vi "动态调用（非模式对话框）串口基本配置对话框.vi"() -> ()   [LabVIEW 2013]
uses:
  <vilib>/Platform/TimedLoop/XDataNode/timing_clust.ctl
  <vilib>/Platform/TimedLoop/XDataNode/nitl_modes.ctl
  <vilib>/Platform/TimedLoop/XDataNode/wakeup.ctl
  <vilib>/Platform/TimedLoop/XDataNode/XDataNode.xnode
  <vilib>/Platform/TimedLoop/XDataNode/XDNodeRunTimeDep.lvlib
panel:
  out "错误输出":errorcluster
  out "应用程序:所有内存中的VI":string[](array[string])
  in  "串口基本配置对话框":bool
  in  "停止":bool
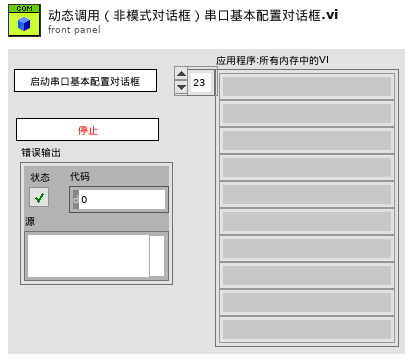
[diagram p1: front panel]
types:
  T1 = typedef "XDNodeRunTimeDep.lvlib/timing_clust.ctl" = cluster{"Expected End [f-1]":u64, "Actual End [f-1]":u64, "Finished Late? [f-1]":bool, "Expected End [i-1]":u64, "Actual End [i-1]":u64, "Finished Late? [i-1]":bool, "Expected Start [i]":u64, "Actual Start [i]":u64, "Expected Start [f]":u64, "Actual Start [f]":u64, "Source Name":string, "Structure Name":string, "Period":i64, "Deadline":i64, "Offset":i64, "Start":i64, "Priority":i32, "Timeout":i32, "Mode":T2, "Wakeup Reason":T3, "Error":errorcluster, "Source Type":string, "Secondary Source Type":string, "Global End Time":u64, "Global Start Time":u64, "Frame Duration":u64, "Iteration Duration":u64, "Assigned CPU":i32, "I/O Scan Engine Mode":u32}
  T2 = typedef "XDNodeRunTimeDep.lvlib/nitl_modes.ctl" = enum32{"No Change", "Process missed periods, maintain original phase", "Discard missed periods, maintain original phase", "Process missed periods, ignore original phase", "Discard missed periods, ignore original phase"}
  T3 = typedef "XDNodeRunTimeDep.lvlib/wakeup.ctl" = enum32{"Normal", "Aborted", "Asynchronous wakeup", "Timing source error", "Timed loop error", "Timeout"}
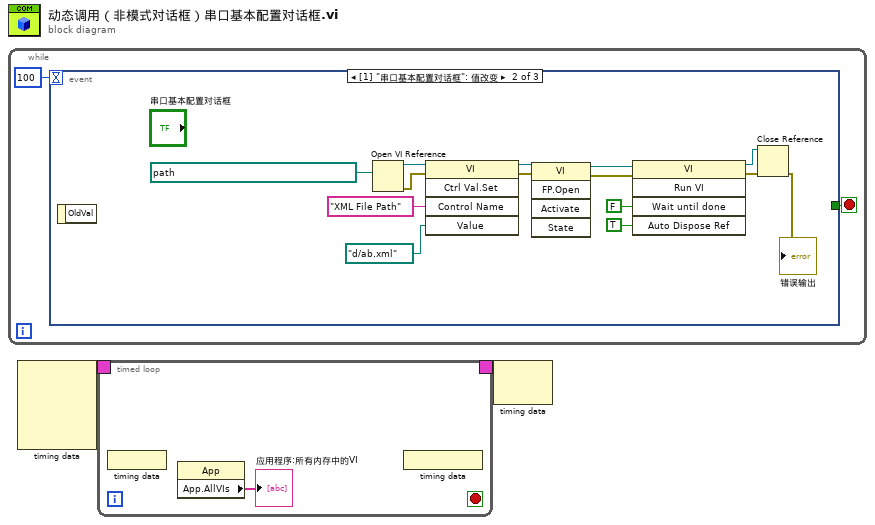
[diagram p0: block diagram]
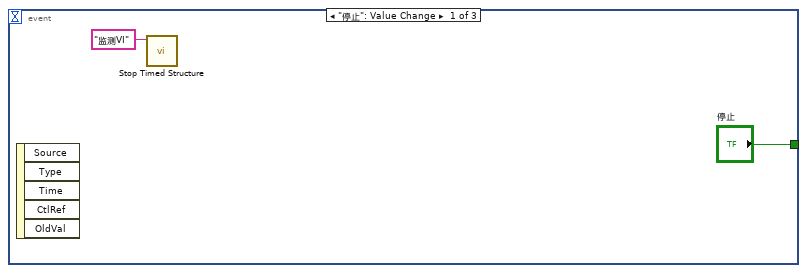
[diagram p2: hidden frame]
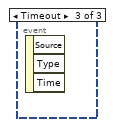
[diagram p3: hidden frame]
diagram:
  n1 = while {
    stop <- w4 stop-if-true
    n2 = event shown="[1] \"串口基本配置对话框\": 值改变" {
      selector: _ -> [_ _ _]
      dyn-events: _ -> [_ _ _]
      timeout: 100 -> [_ _ _]
      tunnel: ["停止" _ _] -> w4
      event "停止": Value Change {
        n3 = event-data() -> ()  [unwired: 1 in, 5 out]
        n4 = call <vilib>:"Stop Timed Structure.vi"("name"="监测VI") -> ()  [unwired: 10 in, 1 out]
      }
      event "串口基本配置对话框": Value Change {
        n5 = event-data() -> ()  [unwired: 1 in, 1 out]
        n6 = Open VI Reference(vi path=path "D:/BOOK/功能块/高级控件/Dlg/串口配置对话框/串口基本配置对话框.vi") -> (vi reference=w19:refnum<vi>, error out=w12:errorcluster)  [unwired: 5 in]
        n7 = invoke class="VI" method="Ctrl Val.Set"(reference=w19, error in=w12, "Control Name"="XML File Path" ("控件名"), "Value"=path "d:/ab.xml" ("XML File Path")) -> (reference out=w10:refnum<vi>, error out=w9:errorcluster)  [unwired: 1 in, 3 out]
        n8 = invoke class="VI" method="FP.Open"(reference=w10, error in=w9) -> (reference out=w8:refnum<vi>, error out=w7:errorcluster)  [unwired: 3 in, 3 out]
        n9 = invoke class="VI" method="Run VI"(reference=w8, error in=w7, "Wait until done"=FALSE ("结束前等待"), "Auto Dispose Ref"=TRUE ("自动销毁引用")) -> (reference out=w14:refnum<vi>, error out=w13:errorcluster)  [unwired: 1 in, 3 out]
        n10 = Close Reference(reference=w14, error in (no error)=w13) -> (error out=→"错误输出":errorcluster)
      }
      event Timeout {
        n11 = event-data() -> ()  [unwired: 1 in, 3 out]
      }
    }
  }
  n12 = node-c288() -> (w2:T1)  [unwired: 4 in]
  n13 = timed-loop {
    timing: w2 -> [_]
    timing-out: [_] -> w1
    stop <- _ stop-if-true
    n14 = node-c288() -> ()  [unwired: 1 in]
    n15 = property class="App"() -> ("App.AllVIs"=→"应用程序:所有内存中的VI":string[])  [unwired: 2 in, 2 out]
    n16 = node-c288() -> ()  [unwired: 1 out]
  }
  n17 = node-c288(w1) -> ()  [unwired: 1 out]
